vi "Get Package ID.vi"(8 "error in (no error)":errorcluster, 11 "Package in":refnum<class "Package.lvclass">) -> (0 "error out":errorcluster, 2 "ID":T1, 3 "Package out":refnum<class "Package.lvclass">)   [LabVIEW 2020, in "neg-pkg.lvlib" / "Package.lvclass"]
uses:
  Package.lvclass
  Package ID.ctl
  Package Type.ctl
  Package.lvclass/Package.ctl
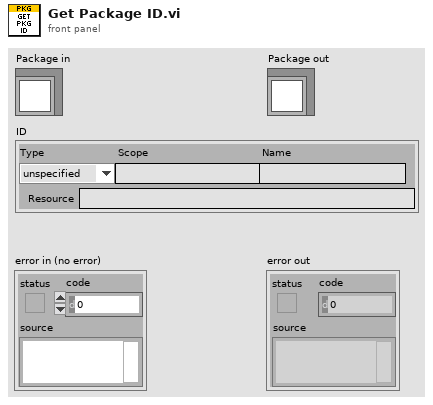
[diagram p1: front panel]
types:
  T1 = typedef "neg-pkg.lvlib/Package.lvclass/Package ID.ctl" = cluster{"Type":T2, "Scope":string, "Name":string, "Resource":string}
  T2 = typedef "neg-pkg.lvlib/Package.lvclass/Package Type.ctl" = enum16{"unspecified", "git"}
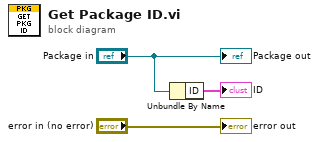
[diagram p0: block diagram]
diagram:
  n1 = Unbundle By Name("Package in") -> ("ID"=→"ID":T1)
  "error out" <- "error in (no error)"
  "Package out" <- "Package in"
